vi "Combined Simulation for v6.0.vi"() -> (1 "Rig Temperatures Cluster":T3, 2 "Line Data (Array of Clusters)":T2(array[cluster]))   [LabVIEW 2018]
panel:
  in  "Line Controls":enum32{"Flowrate", "Temperatures", "Pressures"}(tab)
  in  "Line Flowrate Control":T1 {"Line 5" scale=0.0..10.0; "Line 4" scale=0.0..10.0; "Line 3" scale=0.0..10.0; "Line 2" scale=0.0..10.0; "Line 1" scale=0.0..10.0}
  in  "Temperatures Control":T1 {"Line 5" scale=0.0..10.0; "Line 4" scale=0.0..10.0; "Line 3" scale=0.0..10.0; "Line 2" scale=0.0..10.0; "Line 1" scale=0.0..10.0}
  in  "Pressure Controls":T1 {"Line 5" scale=0.0..10.0; "Line 4" scale=0.0..10.0; "Line 3" scale=0.0..10.0; "Line 2" scale=0.0..10.0; "Line 1" scale=0.0..10.0}
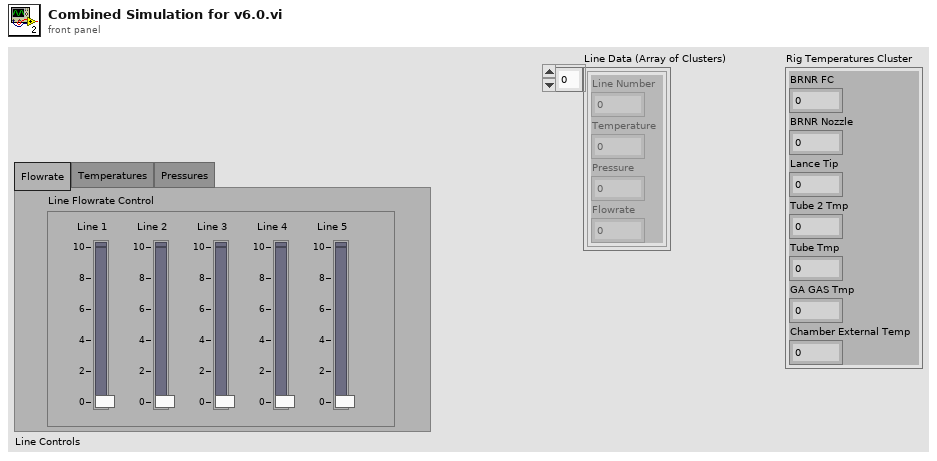
[diagram p1: front panel]
types:
  T1 = cluster{"Line 1":dbl, "Line 2":dbl, "Line 3":dbl, "Line 4":dbl, "Line 5":dbl}
  T2 = cluster{"Line Number":dbl, "Temperature":dbl, "Pressure":dbl, "Flowrate":dbl}[]
  T3 = cluster{"BRNR FC":dbl, "BRNR Nozzle":dbl, "Lance Tip":dbl, "Tube 2 Tmp":dbl, "Tube Tmp":dbl, "GA GAS Tmp":dbl, "Chamber External Temp":dbl}
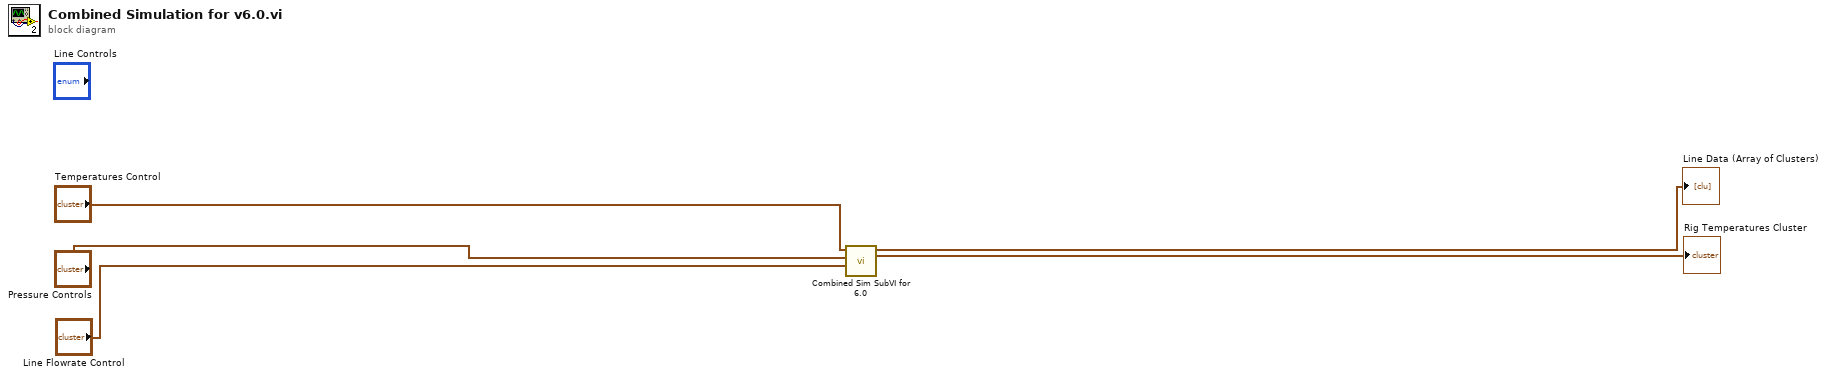
[diagram p0: block diagram]
diagram:
  n1 = call "Combined Sim SubVI for 6.0.vi"("Line Flowrate Control"="Line Flowrate Control", "Pressure Controls"="Pressure Controls", "Temperatures Control"="Temperatures Control") -> ("Cluster"=→"Rig Temperatures Cluster":T3, "Array"=→"Line Data (Array of Clusters)":T2)  [unwired: 7 in]
